vi "Decode Update from Git.vi"(8 "error in (no error)":errorcluster, 11 "Data":variant) -> (0 "error out":errorcluster, 2 "branch name":string, 3 "update from git":bool)   [LabVIEW 2026, in "TALOS.lvlib" / "Guardian.lvlib" / "Guardian.lvclass"]
uses:
  Guardian.lvclass
  TALOS.lvlib
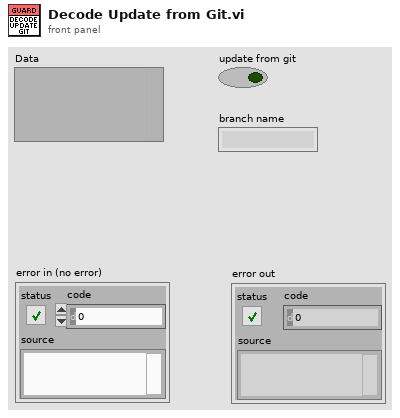
[diagram p1: front panel]
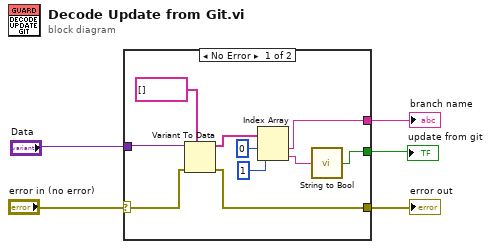
[diagram p0: block diagram]
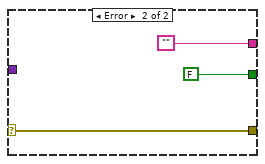
[diagram p2: hidden frame]
diagram:
  n1 = case shown="No Error" "error in (no error)" {
    selector: "error in (no error)" -> [w10 w16]
    tunnel: "Data" -> [w15 _]
    tunnel: [w8 ""] -> w3
    tunnel: [w6 FALSE ("update from git")] -> w2
    tunnel: [w9 w16] -> w1
    frame No Error {
      n2 = Variant To Data(error in=w10, type=string[] [], Variant=w15) -> (data=w13:string[], error out=w9:errorcluster)
      n3 = Index Array(array=w13, index #1=0 ("index"), index #2=1 ("index")) -> (element #1=w8:string, element #2=w7:string)
      n4 = call "String to Bool.vi"("String"=w7) -> ("Boolean"=w6:bool)
    }
    frame Error {
    }
  }
  "branch name" <- w3
  "update from git" <- w2
  "error out" <- w1
